vi "Configure Export Signal.vi"(8 "error in (no error)":errorcluster, 11 "Scope PXI Base CFG in":refnum<class "Scope PXI Base CFG.lvclass">) -> (0 "error out":errorcluster, 3 "Base CFG out":refnum<class "Scope PXI Base CFG.lvclass">)   [LabVIEW 2023, in "Scope PXI Base CFG.lvclass"]
uses:
  Scope PXI Base CFG.lvclass
  <instrlib>/niScope/Controls/niScope exportable signals.ctl
  <instrlib>/niScope/Controls/niScope export destinations.ctl
  Configuration/Configuration JSON/Configuration JSON Base/CFG JSON.lvclass/CFG JSON.ctl
  Scope PXI Base CFG.lvclass/Scope PXI Base CFG.ctl
  42599f19-f05a-4c63-9b72-d5b944f4c65f.vi
  <vilib>/JDP Science/JSONtext/Find Item.vi
  <vilib>/JDP Science/JSONtext/Next JSON Value.vi
  <vilib>/JDP Science/JSONtext/String Subset.vi
  <vilib>/JDP Science/JSONtext/Parsing/Advance past next JSON Value (inlined COPY).vi
  <vilib>/JDP Science/JSONtext/Parsing/Advance past whitespace.vi
  <vilib>/JDP Science/JSONtext/Parsing/Advance past String.vi
  <vilib>/JDP Science/JSONtext/Parsing/Advance past Number.vi
  <vilib>/JDP Science/JSONtext/Parsing/Advance past Line Ending.vi
  <vilib>/JDP Science/JSONtext/Parsing/Parse Full Path or Item Name.vi
  <vilib>/JDP Science/JSONtext/Parsing/Advance past Array.vi
  <vilib>/JDP Science/JSONtext/Parsing/Advance past Object.vi
  <vilib>/JDP Science/JSONtext/support/Error Cluster From Code.vi
  <vilib>/JDP Science/JSONtext/Offset/Find Item Locations by Path.vi
  <vilib>/JDP Science/JSONtext/JSON text to Variant.vi
  <vilib>/Utility/error.llb/Error Cluster From Error Code.vi
  <vilib>/JDP Science/JSONtext/LVClass Serializer/JSONtext LVClass Serializer.lvclass
  <vilib>/ErrorRing/Error Ring.xnode
  Configuration/Configuration JSON/Configuration JSON Base/CFG JSON.lvclass
  D:/git/HAL/HAL GOOP4/Configuration/Configuration JSON/Configuration JSON Base/CFG JSON.lvclass
  D:/git/HAL/HAL GOOP4/Interfaces/IConfigure/IConfigure.lvclass
  D:/git/HAL/HAL GOOP4/Scope/Scope PXI/Base CFG/Scope PXI Base CFG.lvclass
  D:/git/HAL/HAL GOOP4/Interfaces/IConfigure Scope/IConfigure Scope.lvclass
panel:
  out "signal":T1 caption="signal (Start Trigger)" items=["None"=0, "Start Trigger"=2, "Advance Trigger"=5, "Reference Trigger"=1, "End of Record Event"=4, "End of Acquisition Event"=3, "Ready for Start Event"=7, "Ready for Advance Event"=6, "Ready for Reference Event"=10, "Reference Clock"=100, "Sample Clock"=101, "5 Volt Power"=13]
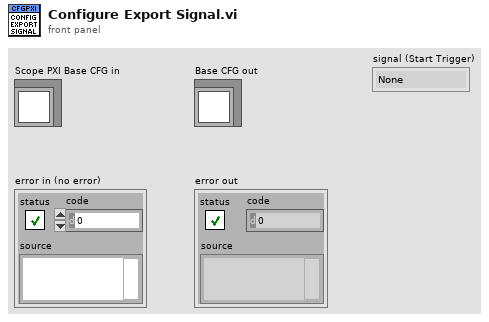
[diagram p1: front panel]
types:
  T1 = typedef "niScope exportable signals.ctl" = u16
  T2 = typedef "niScope export destinations.ctl" = string
  T3 = cluster{"Signal Identifier":string, "Signal":string, "Output Terminal":T2}
  T4 = typedef "LVStringsAndValuesArrayTypeDef_U16.ctl" = cluster{"String":string, "Value":u16}[]
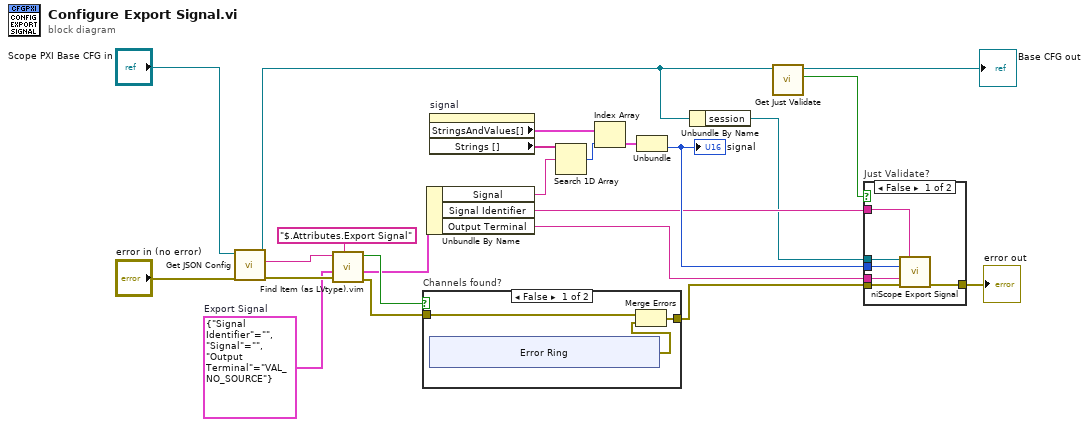
[diagram p0: block diagram]
diagram:
  w12 = T3 {"Signal Identifier"="", "Signal"="", "Output Terminal"="VAL_NO_SOURCE"}  # Export Signal
  n1 = call "Get JSON Config.vi"("error in (no error)"="error in (no error)", "CFG Base in"="Scope PXI Base CFG in") -> ("error out"=w22:errorcluster, "<JSON>Config>"=w21:string, "CFG Base out"=w14:refnum<class "Scope PXI Base CFG.lvclass">)  [unwired: 7 in]
  n2 = call "Find Item (as LVtype).vim"("$Path or Item Name"="$.Attributes.Export Signal", "error in (no error)"=w22, "Data Type and Default Value"=w12, "JSON"=w21) -> ("error out"=w11:errorcluster, "Data"=w7:T3, "Found"=w10:bool)  [unwired: 4 in, 1 out]
  n3 = case "Channels found?" shown="False" w10 {
    tunnel: [w26 w32] -> w9
    tunnel: w11 -> [w24 w32]
    frame False {
      n4 = xnode "Error Ring"() -> ("error out"=w25:errorcluster)
      n5 = Merge Errors(w24, w25) -> (w26:errorcluster)
    }
    frame True {
    }
  }
  n6 = Unbundle By Name(w7) -> ("Signal"=w6:string, "Signal Identifier"=w5:string, "Output Terminal"=w4:T2)
  n7 = property on="signal" class="Ring (strict)"() -> ("StringsAndValues[]"=w19:T4, "Strings []"=w20:string[])  [unwired: 2 in, 2 out]
  n8 = Search 1D Array(1D array=w20, element=w6) -> (index of element=w18:i32)  [unwired: 1 in]
  n9 = Index Array(array=w19, index=w18) -> (element=w17:cluster{"String":string, "Value":u16})
  n10 = Unbundle(w17) -> ("Value"=w8:u16)  [unwired: 1 out]
  "signal" <- w8
  n11 = Unbundle By Name(w14) -> ("session"=w3:refnum<k15>)
  n12 = call "Get Just Validate.vi"("CFG JSON Base in"=w14) -> ("Just Validate"=w1:bool, "CFG JSON Base out"=→"Base CFG out":refnum<class "Scope PXI Base CFG.lvclass">)  [unwired: 8 in, 1 out]
  n13 = case "Just Validate?" shown="False" w1 {
    tunnel: w3 -> [w38 _]
    tunnel: [w37 w39] -> w16
    tunnel: w9 -> [w36 w39]
    tunnel: w8 -> [w35 _]
    tunnel: w5 -> [w34 _]
    tunnel: w4 -> [w33 _]
    frame False {
      n14 = call <instrlib>:"niScope Export Signal.vi"("instrument handle"=w38, "signal identifier"=w34, "signal"=w35, "output terminal"=w33, "error in"=w36) -> ("error out"=w37:errorcluster)  [unwired: 9 in, 1 out]
    }
    frame True {
    }
  }
  "error out" <- w16
